vi "Dialog Normal.vi"(8 "error in (no error)":errorcluster, 9 "Caption 2(CANCEL)":string="CANCEL", 10 "Caption 1(OK)":string="OK", 11 "Message":string) -> (0 "error out":errorcluster, 2 "Button 2 pressed":bool, 3 "Button 1 pressed":bool)   [LabVIEW 2016]
panel:
  in  "Button 2":bool
  in  "Button 1":bool
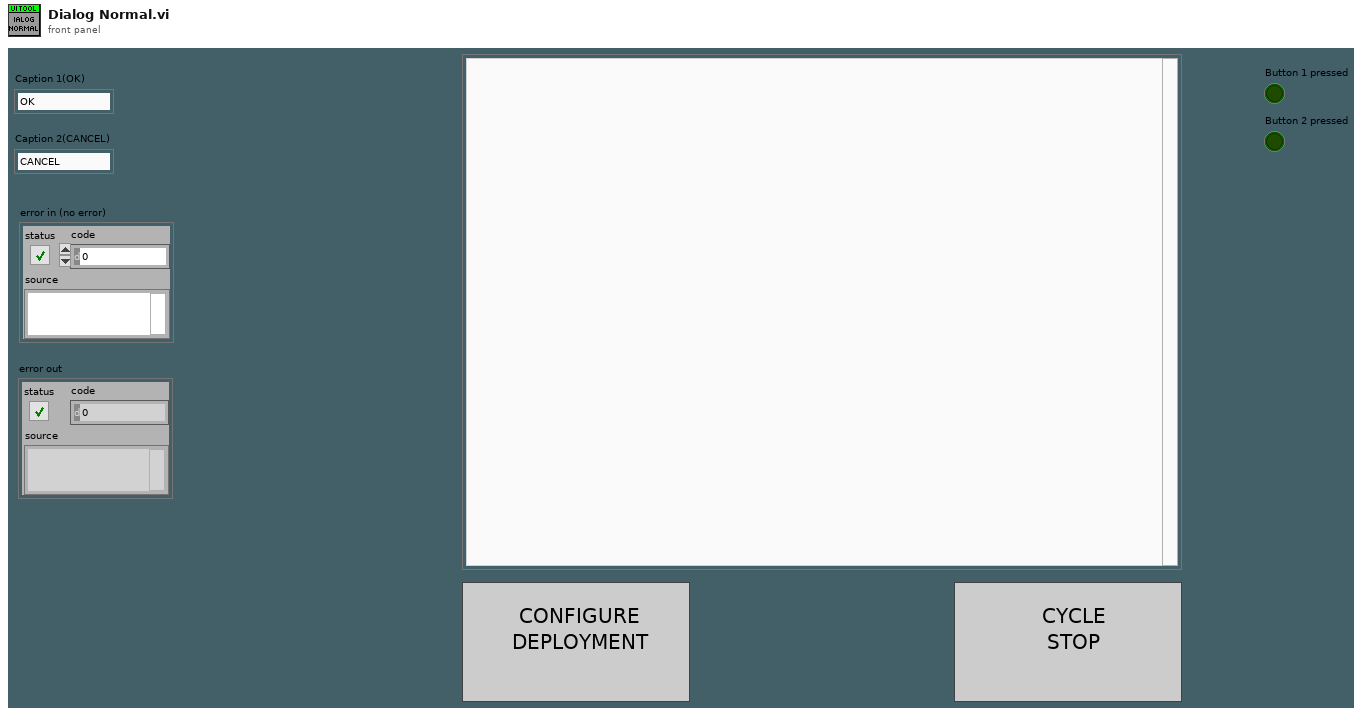
[diagram p1: front panel]
types:
  T1 = enum32{"Invalid", "Default", "Floating", "Floating/Auto-Hide", "Modal"}
  T2 = enum32{"invalid app kind", "Development System", "Run Time System", "Student Edition", "Embedded LabVIEW", "Evaluation", "Custom"}
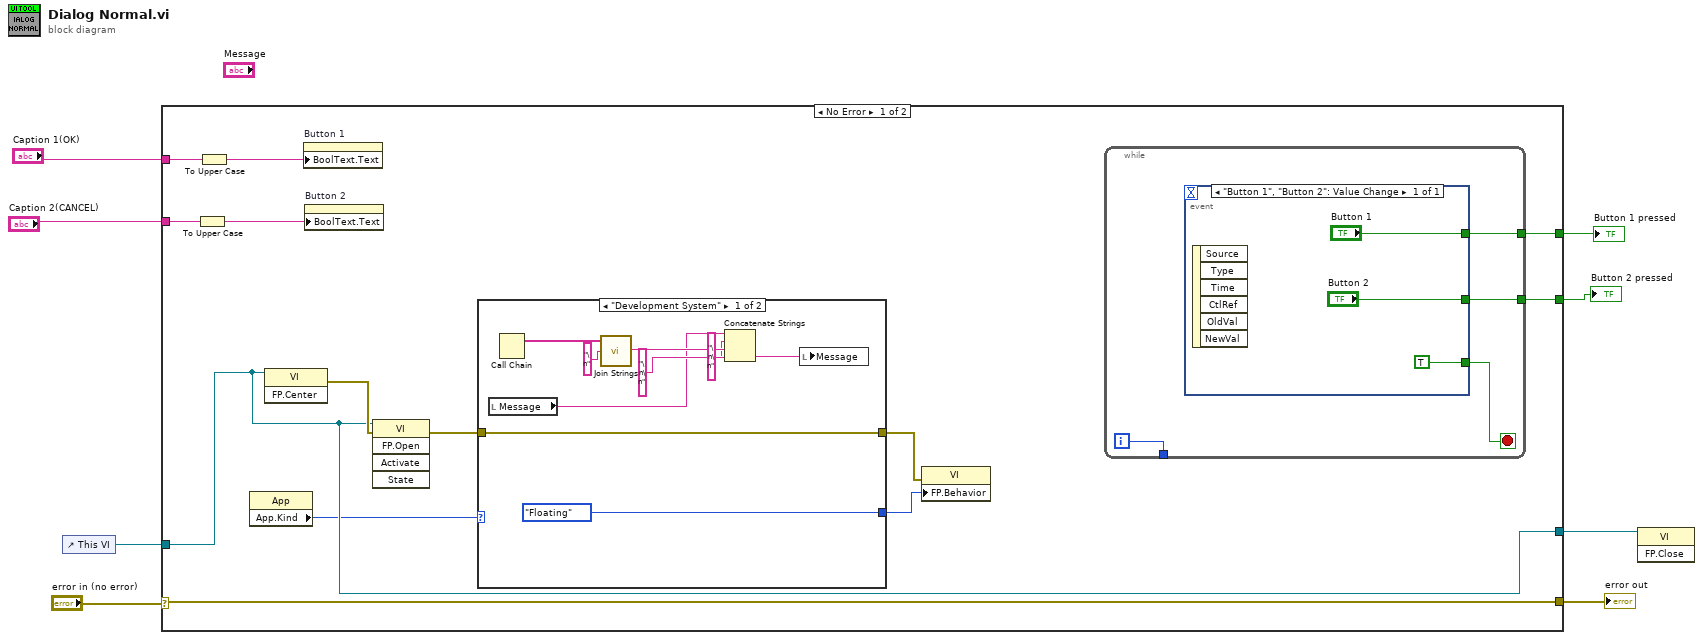
[diagram p0: block diagram]
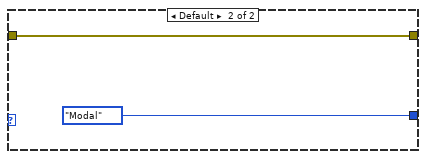
[diagram p2: hidden frame]
diagram:
  n1 = control-ref of="This VI"() -> (w1:refnum<vi>)
  n2 = case shown="No Error" "error in (no error)" {
    selector: "error in (no error)" -> [w21 w41]
    tunnel: "Caption 1(OK)" -> [w12 _]
    tunnel: "Caption 2(CANCEL)" -> [w13 _]
    tunnel: [w21 w41] -> w5
    tunnel: [w20 _] -> w4
    tunnel: [w19 _] -> w3
    tunnel: [w14 w40] -> w2
    tunnel: w1 -> [w14 w40]
    frame No Error {
      n3 = To Upper Case(1:w13) -> (0:w10:string)
      n4 = To Upper Case(1:w12) -> (0:w11:string)
      n5 = property class="App"() -> ("App.Kind"=w9:T2)  [unwired: 2 in, 2 out]
      n6 = invoke class="VI" method="FP.Center"(reference=w14) -> (error out=w18:errorcluster)  [unwired: 2 in, 2 out]
      n7 = property on="Button 1" class="Bool"("BoolText.Text"=w11) -> ()  [unwired: 2 in, 2 out]
      n8 = property on="Button 2" class="Bool"("BoolText.Text"=w10) -> ()  [unwired: 2 in, 2 out]
      n9 = invoke class="VI" method="FP.Open"(reference=w14, error in=w18) -> (error out=w15:errorcluster)  [unwired: 3 in, 4 out]
      n10 = case shown="\"Development System\"" w9 {
        tunnel: [T1."Floating" ("Front Panel Window:Behavior") T1."Modal" ("Front Panel Window:Behavior")] -> w17
        tunnel: [w36 w38] -> w16
        tunnel: w15 -> [w36 w38]
        frame "Development System" {
          n11 = local read "Message"() -> (w30:string)
          n12 = Call Chain() -> (call chain=w34:string[])
          n13 = call <vilib>:"Join Strings.vi"("Separator (,)"="\n", "Strings In"=w34) -> ("String"=w33:string)  [unwired: 1 in]
          n14 = Concatenate Strings(w30, "\n\n" ("string"), w33, "\n\n" ("string")) -> (w31:string)
          n15 = local write "Message"(w31) -> ()
        }
        frame Default {
        }
      }
      n16 = property class="VI"(error in=w16, "FP.Behavior"=w17) -> ()  [unwired: 1 in, 2 out]
      n17 = while {
        tunnel: [w25] -> w20
        tunnel: [w24] -> w19
        tunnel: [w22] -> _
        i -> [w22]
        stop <- w23 stop-if-true
        n18 = event shown="[0] \"Button 1\", \"Button 2\": Value Change" {
          selector: _ -> [_]
          dyn-events: _ -> [_]
          timeout: _ -> [_]
          tunnel: ["Button 1"] -> w25
          tunnel: ["Button 2"] -> w24
          tunnel: [TRUE] -> w23
          event "Button 1", "Button 2": Value Change {
            n19 = event-data() -> ()  [unwired: 1 in, 6 out]
          }
        }
      }
    }
    frame Error {
    }
  }
  "error out" <- w5
  "Button 1 pressed" <- w4
  "Button 2 pressed" <- w3
  n20 = invoke class="VI" method="FP.Close"(reference=w2) -> ()  [unwired: 2 in, 3 out]
